vi "cblas drot.vi"(5 "n":i32=-1, 6 "incy":i32=1, 7 "incx":i32=1, 8 "s":dbl, 9 "c":dbl=1.0, 10 "y in":dbl[](array[numeric]), 11 "x in":dbl[](array[numeric])) -> (0 "error":i32, 2 "y out":dbl[](array[numeric]), 3 "x out":dbl[](array[numeric]))   [LabVIEW 2017, in "NI_AALBLAS.lvlib"]
uses:
  NI_AALBLAS.lvlib
  lvblas.dll
panel:
  # "void cblas_drot(n, *x, incx, *y, incy, c, s)"
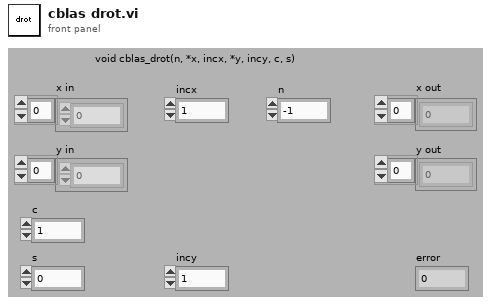
[diagram p1: front panel]
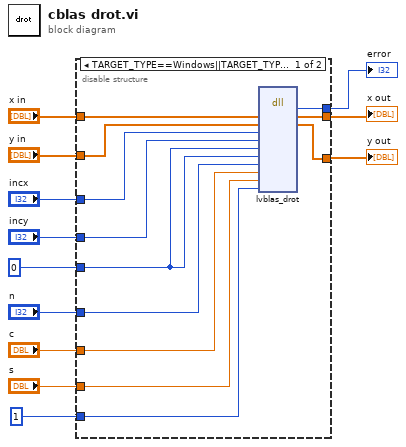
[diagram p0: block diagram]
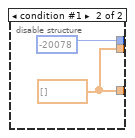
[diagram p2: hidden frame]
diagram:
  n1 = disable-structure shown="TARGET_TYPE==Windows||TARGET_TYPE==Unix||TARGET_TYPE==RT||TARGET_TYPE==Mac" {
    disable-tunnel: "x in" -> [w24 _]
    disable-tunnel: "y in" -> [w23 _]
    disable-tunnel: "n" -> [w22 _]
    disable-tunnel: [w21 -20078] -> w9
    disable-tunnel: 0 -> [w20 _]
    disable-tunnel: [w19 w25] -> w7
    disable-tunnel: [w18 w25] -> w6
    disable-tunnel: "c" -> [w17 _]
    disable-tunnel: "s" -> [w16 _]
    disable-tunnel: "incx" -> [w15 _]
    disable-tunnel: "incy" -> [w14 _]
    disable-tunnel: 1 -> [w13 _]
    frame condition #0 (active) {
      n2 = dll-call lib="C:/Program Files/National Instruments/LabVIEW 2017/resource/lvblas.*" fn="lvblas_drot" ("CBLAS.dll:DotProdH")("X"=w24, "Y"=w23, "IncX"=w15, "IncY"=w14, "startX"=w20, "startY"=w20, "N"=w22, "c"=w17, "s"=w16, "check"=w13) -> ("error"=w21:i32, "X"=w19:dbl[], "Y"=w18:dbl[])  [unwired: 11 in, 2 out]
    }
    frame condition #1 {
      w25 = dbl[] []
    }
  }
  "error" <- w9
  "x out" <- w7
  "y out" <- w6
